vi "Test.vi"() -> ()   [LabVIEW 2011, in "Valve Controller.lvclass"]
uses:
  Valve Controller.lvclass
  Valves.ctl
  Status.ctl
  PID/Controls/Valve Type.ctl
  INL Valve Controller/INL Valve Controller.lvclass
panel:
  in  "Valve Type":T1
  out "status out 2":T2 items=["Closed", "Open"]
  out "valves out":T3=7 items=["Valve 1"=1, "Valve 2"=2, "Valve 3"=3, "Valve 4"=4, "Valve 5"=5, "Valve 6"=6, "Valve 7"=7]
  in  "valves in":T3=7 items=["Valve 1"=1, "Valve 2"=2, "Valve 3"=3, "Valve 4"=4, "Valve 5"=5, "Valve 6"=6, "Valve 7"=7]
  out "status out":T2 items=["Closed", "Open"]
  out "Valves out":T3=7 items=["Valve 1"=1, "Valve 2"=2, "Valve 3"=3, "Valve 4"=4, "Valve 5"=5, "Valve 6"=6, "Valve 7"=7]
  in  "status in":T2 items=["Closed", "Open"]
  in  "valve in":T3 items=["Valve 1"=1, "Valve 2"=2, "Valve 3"=3, "Valve 4"=4, "Valve 5"=5, "Valve 6"=6, "Valve 7"=7]
  out "error out":errorcluster
  in  "error in (no error)":errorcluster
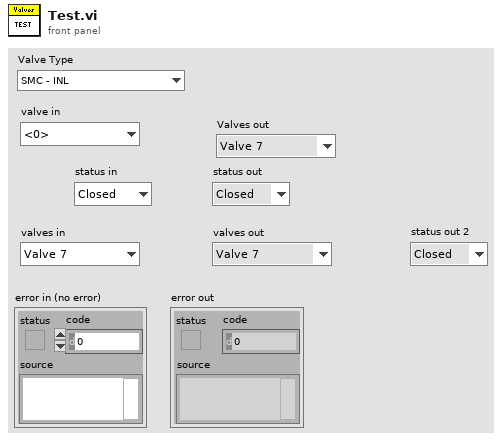
[diagram p1: front panel]
types:
  T1 = typedef "Valve Type.ctl" = enum16{"SMC - INL"}
  T2 = typedef "Valve Controller.lvclass/Status.ctl" = u16
  T3 = typedef "Valve Controller.lvclass/Valves.ctl" = u16
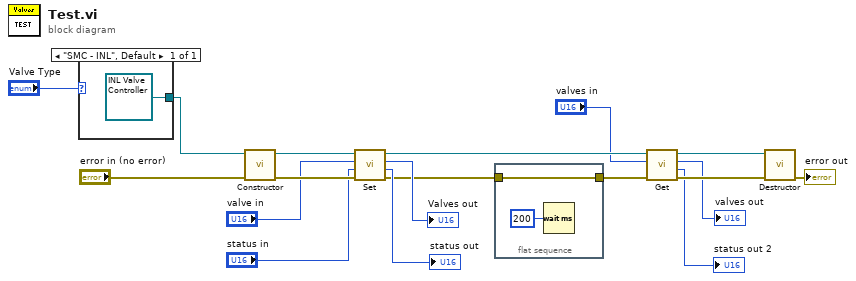
[diagram p0: block diagram]
diagram:
  n1 = case shown="\"SMC - INL\", Default" "Valve Type" {
    tunnel: [refnum<class "INL Valve Controller.lvclass"> refnum ("INL Valve Controller.lvclass")] -> w1
    frame "SMC - INL", Default {
    }
  }
  n2 = call-dynamic "Constructor.vi"("error in (no error)"="error in (no error)", "INL Valve Controller in"=w1) -> ("error out"=w17:errorcluster, "INL Valve Controller out"=w16:refnum<class "INL Valve Controller.lvclass">)  [unwired: 7 in, 1 out]
  n3 = call-dynamic "Set.vi"("error in (no error)"=w17, "status in"="status in", "valve in"="valve in", "INL Valve Controller in"=w16) -> ("error out"=w4:errorcluster, "status out"=→"status out":T2, "Valve out"=→"Valves out":T3, "INL Valve Controller out"=w10:refnum<class "INL Valve Controller.lvclass">)  [unwired: 4 in]
  n4 = flat-sequence {
    tunnel: w4 -> [w21]
    tunnel: [w21] -> w3
    frame #0 {
      n5 = Wait (ms)(milliseconds to wait=u32 200) -> ()  [unwired: 1 out]
    }
  }
  n6 = call-dynamic "Get.vi"("error in (no error)"=w3, "valve in"="valves in", "INL Valve Controller in"=w10) -> ("error out"=w7:errorcluster, "status out"=→"status out 2":T2, "valve out"=→"valves out":T3, "INL Valve Controller out"=w8:refnum<class "INL Valve Controller.lvclass">)  [unwired: 5 in]
  n7 = call-dynamic "Destructor.vi"("error in (no error)"=w7, "INL Valve Controller in"=w8) -> ("error out"=→"error out":errorcluster)  [unwired: 8 in, 1 out]
